vi "Set Active Cursor from Table.vi"(9 "Point":cluster{"horizontal":i32, "vertical":i32}, 10 "Refnums for Resizing and Alignment":T4, 11 "Display State In":T1={"Graph Visible Items"={"Plot Legend"=FALSE, "Scale Legend"=FALSE, "Graph Palette"=FALSE, "Cursor Legend"=FALSE, "X Scrollbar"=FALSE}, "View Table"=FALSE, "Table Visible Items"={"Vertical Scrollbar"=FALSE, "Horizontal Scrollbar"=FALSE, "Row Headers"=FALSE, "Column Headers"=FALSE, "Vertical Lines"=FALSE, "Horizontal Lines"=FALSE}, "Header Font"={"Font Name"="", "Size"=0, "Bold"=FALSE, "Italic"=FALSE, "Underline"=FALSE, "Strikeout"=FALSE, "Color"=0}, "Cell Font"={"Font Name"="", "Size"=0, "Bold"=FALSE, "Italic"=FALSE, "Underline"=FALSE, "Strikeout"=FALSE, "Color"=0}, "Description and Tip..."={"Description"="", "Tip"=""}, "Moveable Splitter Position"=0, "Measurement Cursor Configuration"={"relative to t0"={"enable relative time"=FALSE, "Relative times (DT)"=[], "color"=0}, "range"={"enable range"=FALSE, "T1"=0.0, "T2"=0.0, "Fixed interval (T2-T1)"=0.0, "T1 color"=0, "T2 color"=0, "enable shading"=FALSE}, "periodic"={"enable periodic"=FALSE, "First event (E1)"=0.0, "Number events (Ei)"=0, "Event spacing (s)"=0.0, "First color"=0, "Events color"=0}, "absolute timestamp"={"enable absolute"=FALSE, "Timestamps (TS)"=[], "color"=0}}, "X Increment"=0.0, "X Scale"={"Label Visible"=FALSE, "Label Text"="", "Time Mode"=enum."Relative", "Format String"=""}, "Y Scale"={"Label Visible"=FALSE, "Label Text"="", "Scaling"=enum."Engineering Units", "Format String"=""}, "Colors"={"background"=16777215, "major grid"=8355711, "minor grid"=12632256, "font"=0}, "Cursors"={"List"=[], "Tags"=[]}, "Plots"=[], "Plot Color Wheel"=[3381759, 32768, 982784, 4375295, 13827953, 13457919, 16757522, 4343295, 16728758, 12095254], "registered user events"=variant} caption="State") -> (3 "Display State Out":T1={"Graph Visible Items"={"Plot Legend"=FALSE, "Scale Legend"=FALSE, "Graph Palette"=FALSE, "Cursor Legend"=FALSE, "X Scrollbar"=FALSE}, "View Table"=FALSE, "Table Visible Items"={"Vertical Scrollbar"=FALSE, "Horizontal Scrollbar"=FALSE, "Row Headers"=FALSE, "Column Headers"=FALSE, "Vertical Lines"=FALSE, "Horizontal Lines"=FALSE}, "Header Font"={"Font Name"="", "Size"=0, "Bold"=FALSE, "Italic"=FALSE, "Underline"=FALSE, "Strikeout"=FALSE, "Color"=0}, "Cell Font"={"Font Name"="", "Size"=0, "Bold"=FALSE, "Italic"=FALSE, "Underline"=FALSE, "Strikeout"=FALSE, "Color"=0}, "Description and Tip..."={"Description"="", "Tip"=""}, "Moveable Splitter Position"=0, "Measurement Cursor Configuration"={"relative to t0"={"enable relative time"=FALSE, "Relative times (DT)"=[], "color"=0}, "range"={"enable range"=FALSE, "T1"=0.0, "T2"=0.0, "Fixed interval (T2-T1)"=0.0, "T1 color"=0, "T2 color"=0, "enable shading"=FALSE}, "periodic"={"enable periodic"=FALSE, "First event (E1)"=0.0, "Number events (Ei)"=0, "Event spacing (s)"=0.0, "First color"=0, "Events color"=0}, "absolute timestamp"={"enable absolute"=FALSE, "Timestamps (TS)"=[], "color"=0}}, "X Increment"=0.0, "X Scale"={"Label Visible"=FALSE, "Label Text"="", "Time Mode"=enum."Relative", "Format String"=""}, "Y Scale"={"Label Visible"=FALSE, "Label Text"="", "Scaling"=enum."Engineering Units", "Format String"=""}, "Colors"={"background"=16777215, "major grid"=8355711, "minor grid"=12632256, "font"=0}, "Cursors"={"List"=[], "Tags"=[]}, "Plots"=[], "Plot Color Wheel"=[3381759, 32768, 982784, 4375295, 13827953, 13457919, 16757522, 4343295, 16728758, 12095254], "registered user events"=variant} caption="State")   [LabVIEW 2017, in "Waveforms with Cursors.xctl"]
doc: "Make selected row active cursor and highlight cursor row in table."
uses:
  <vilib>/addons/_XControls/Waveforms with Cursors/Waveforms with Cursors.xctl
  <vilib>/addons/_XControls/Waveforms with Cursors/Controls/State.ctl
  <vilib>/Utility/miscctls.llb/LVFontTypeDef.ctl
  <vilib>/addons/_XControls/Waveforms with Cursors/Controls/Waveform Cursor Configuration.ctl
  <vilib>/addons/_XControls/Waveforms with Cursors/Controls/Refnums Typedef.ctl
  <vilib>/Utility/miscctls.llb/LVPositionTypeDef.ctl
  <vilib>/Utility/miscctls.llb/LVRowAndColumnTypeDef.ctl
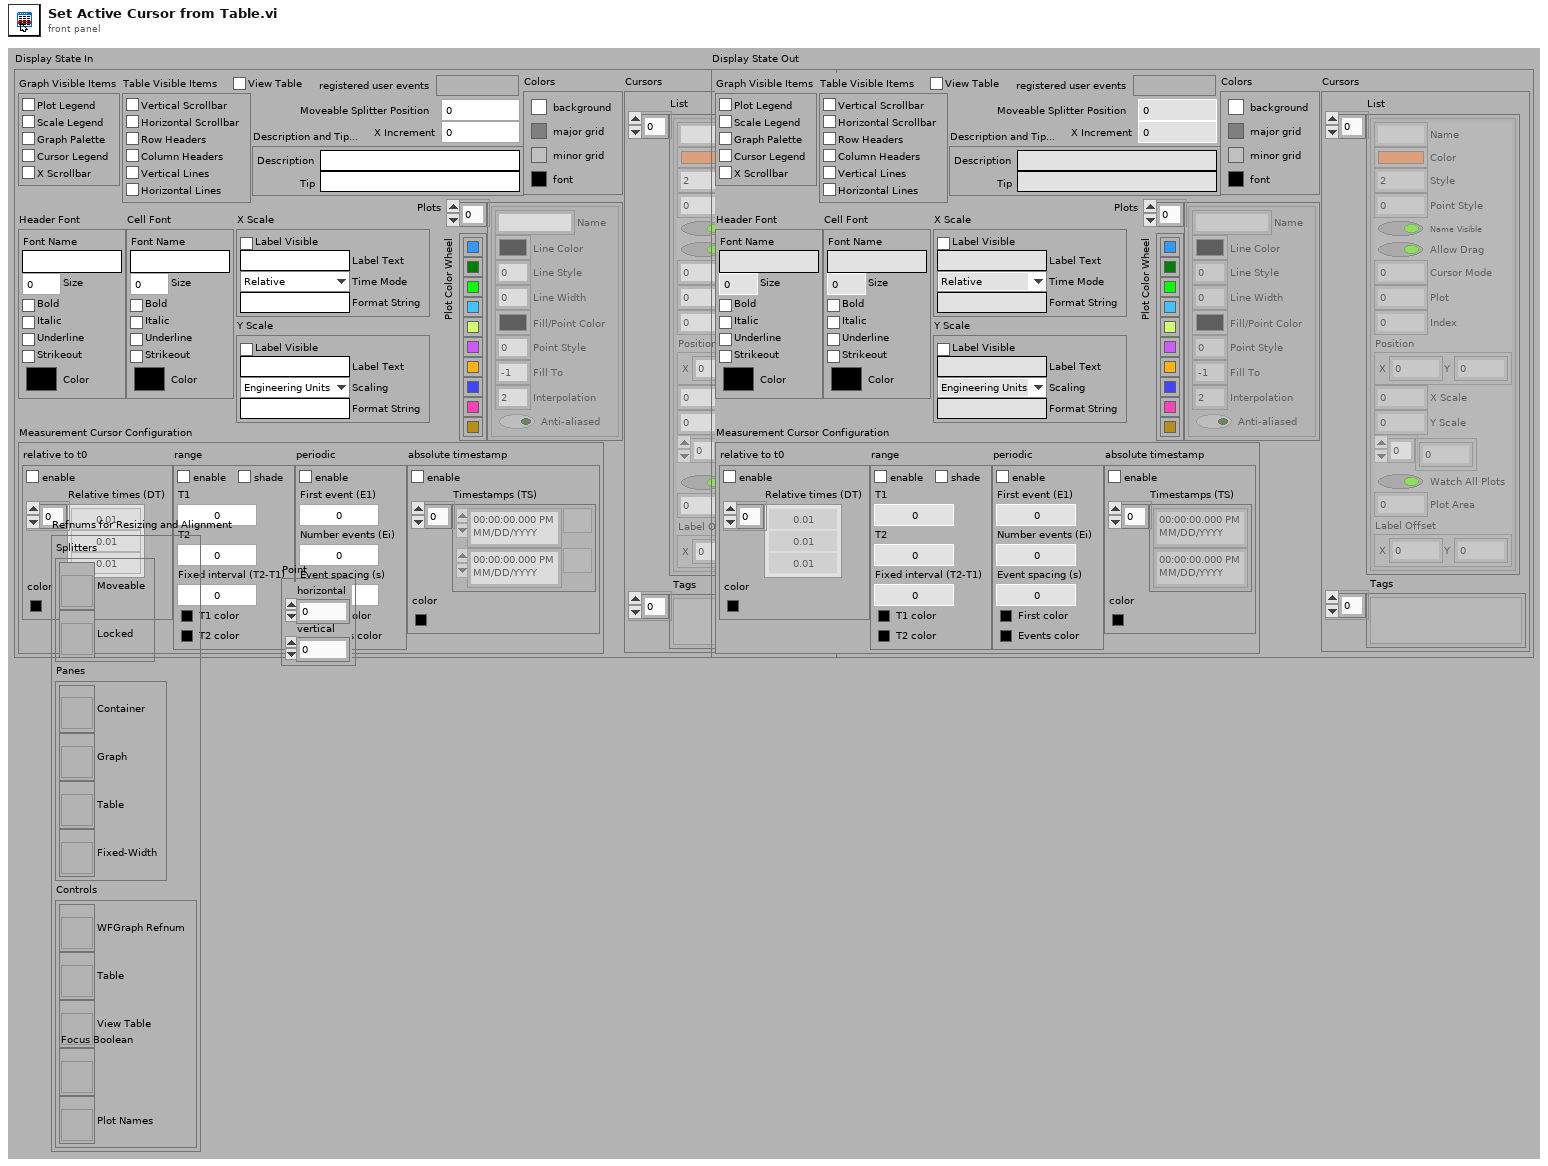
[diagram p1: front panel]
types:
  T1 = typedef "Waveforms with Cursors.xctl/State.ctl" = cluster{"Graph Visible Items":cluster{"Plot Legend":bool, "Scale Legend":bool, "Graph Palette":bool, "Cursor Legend":bool, "X Scrollbar":bool}, "View Table":bool, "Table Visible Items":cluster{"Vertical Scrollbar":bool, "Horizontal Scrollbar":bool, "Row Headers":bool, "Column Headers":bool, "Vertical Lines":bool, "Horizontal Lines":bool}, "Header Font":T2, "Cell Font":T2, "Description and Tip...":cluster{"Description":string, "Tip":string}, "Moveable Splitter Position":i32, "Measurement Cursor Configuration":T3, "X Increment":dbl, "X Scale":cluster{"Label Visible":bool, "Label Text":string, "Time Mode":enum16{"Relative", "Absolute"}, "Format String":string}, "Y Scale":cluster{"Label Visible":bool, "Label Text":string, "Scaling":enum16{"Engineering Units", "Voltage"}, "Format String":string}, "Colors":cluster{"background":u32, "major grid":u32, "minor grid":u32, "font":u32}, "Cursors":cluster{"List":cluster{"Name":string, "Color":u32, "Style":i32, "Point Style":u8, "Name Visible":bool, "Allow Drag":bool, "Cursor Mode":u32, "Plot":i32, "Index":i32, "Position":cluster{"X":dbl, "Y":dbl}, "X Scale":u32, "Y Scale":u32, "Watch Plots":i32[], "Watch All Plots":bool, "Plot Area":i32, "Label Offset":cluster{"X":dbl, "Y":dbl}}[], "Tags":variant[]}, "Plots":cluster{"Name":string, "Line Color":u32, "Line Style":u8, "Line Width":u8, "Fill/Point Color":u32, "Point Style":u8, "Fill To":i16, "Interpolation":u8, "Anti-aliased":bool}[], "Plot Color Wheel":u32[], "registered user events":variant}
  T2 = typedef "LVFontTypeDef.ctl" = cluster{"Font Name":string, "Size":u16, "Bold":bool, "Italic":bool, "Underline":bool, "Strikeout":bool, "Color":u32}
  T3 = typedef "Waveforms with Cursors.xctl/Waveform Cursor Configuration.ctl" = cluster{"relative to t0":cluster{"enable relative time":bool, "Relative times (DT)":dbl[], "color":u32}, "range":cluster{"enable range":bool, "T1":dbl, "T2":dbl, "Fixed interval (T2-T1)":dbl, "T1 color":u32, "T2 color":u32, "enable shading":bool}, "periodic":cluster{"enable periodic":bool, "First event (E1)":dbl, "Number events (Ei)":i32, "Event spacing (s)":dbl, "First color":u32, "Events color":u32}, "absolute timestamp":cluster{"enable absolute":bool, "Timestamps (TS)":timestamp[], "color":u32}}
  T4 = typedef "Waveforms with Cursors.xctl/Refnums Typedef.ctl" = cluster{"Splitters":cluster{"Moveable":refnum<vi>, "Locked":refnum<vi>}, "Panes":cluster{"Container":refnum<vi>, "Graph":refnum<vi>, "Table":refnum<vi>, "Fixed-Width":refnum<vi>}, "Controls":cluster{"WFGraph Refnum":refnum<vi>, "Table":refnum<vi>, "View Table":refnum<vi>, "Focus Boolean":refnum<vi>, "Plot Names":refnum<vi>}}
  T5 = typedef "LVPositionTypeDef.ctl" = cluster{"Left":i32, "Top":i32}
  T6 = typedef "LVRowAndColumnTypeDef.ctl" = cluster{"Row":i32, "Column":i32}
  T7 = cluster{"Name":string, "Color":u32, "Style":i32, "Point Style":u8, "Name Visible":bool, "Allow Drag":bool, "Cursor Mode":u32, "Plot":i32, "Index":i32, "Position":cluster{"X":dbl, "Y":dbl}, "X Scale":u32, "Y Scale":u32, "Watch Plots":i32[], "Watch All Plots":bool, "Plot Area":i32, "Label Offset":cluster{"X":dbl, "Y":dbl}}[]
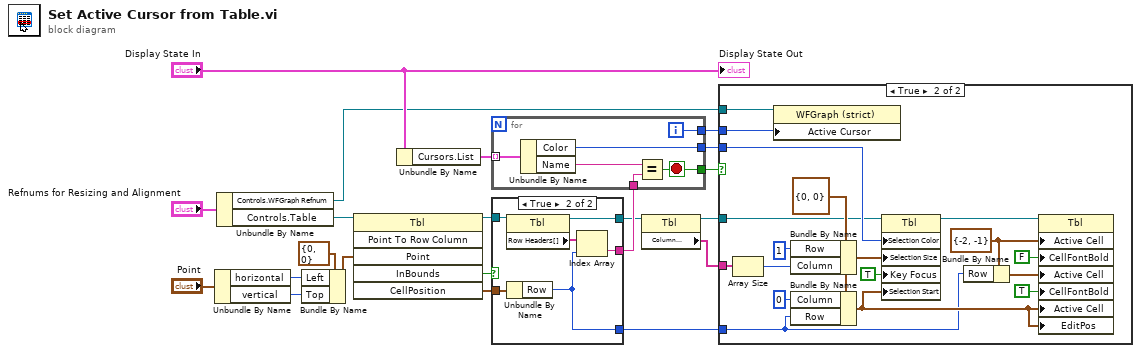
[diagram p0: block diagram]
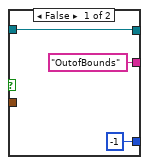
[diagram p3: hidden frame]
diagram:
  n1 = Unbundle By Name("Point") -> ("horizontal"=w9:i32, "vertical"=w8:i32)
  n2 = Unbundle By Name("Refnums for Resizing and Alignment") -> ("Controls.WFGraph Refnum"=w7:refnum<vi>, "Controls.Table"=w16:refnum<vi>)
  n3 = Bundle By Name(cluster=T5 {"Left"=0, "Top"=0} ("Point"), "Left"=w9, "Top"=w8) -> (w10:T5)
  n4 = invoke class="Tbl" method="Point To Row Column"(reference=w16, "Point"=w10) -> (reference out=w17:refnum<vi>, "InBounds"=w15:bool, "CellPosition"=w1:T6)  [unwired: 4 in, 3 out]
  n5 = Unbundle By Name("Display State In") -> ("Cursors.List"=w18:T7)
  n6 = case shown="True" w15 {
    tunnel: w1 -> [_ w30]
    tunnel: w17 -> [w23 w29]
    tunnel: ["OutofBounds" w27] -> w19
    tunnel: [w23 w26] -> w4
    tunnel: [-1 ("Row") w25] -> w6
    frame False {
    }
    frame True {
      n7 = property class="Tbl"(reference=w29) -> (reference out=w26:refnum<vi>, "Row Headers[]"=w28:string[])  [unwired: 1 in, 1 out]
      n8 = Unbundle By Name(w30) -> ("Row"=w25:i32)
      n9 = Index Array(array=w28, index=w25) -> (element=w27:string)
    }
  }
  n10 = for {
    tunnel: w18 -> [w33] mode=indexing
    tunnel: w19 -> [w36]
    tunnel: [w35] -> w20
    tunnel: [w34] -> w21
    tunnel: [w32] -> w5
    i -> [w34]
    stop <- w35 stop-if-true
    n11 = Unbundle By Name(w33) -> ("Color"=w32:u32, "Name"=w31:string)
    n12 = Equal?(x=w31, y=w36) -> (x = y?=w35:bool)
  }
  n13 = property class="Tbl"(reference=w4) -> (reference out=w3:refnum<vi>, "Column Headers[]"=w2:string[])  [unwired: 1 in, 1 out]
  n14 = case shown="True" w20 {
    tunnel: w7 -> [_ w54]
    tunnel: w21 -> [_ w53]
    tunnel: w6 -> [_ w37]
    tunnel: w5 -> [_ w48]
    tunnel: w3 -> [_ w47]
    tunnel: w2 -> [_ w46]
    frame False {
    }
    frame True {
      w42 = T6 {"Row"=-2, "Column"=-1} ("Active Cell:Active Cell")
      w49 = T6 {"Row"=0, "Column"=0} ("Selection Size")
      n15 = Array Size(array=w46) -> (size(s)=w44:i32)
      n16 = property class="WFGraph (strict)"(reference=w54, "Active Cursor"=w53) -> ()  [unwired: 1 in, 2 out]
      n17 = Bundle By Name(cluster=w49, "Row"=1, "Column"=w44) -> (w51:T6)
      n18 = Bundle By Name(cluster=w49, "Column"=0, "Row"=w37) -> (w38:T6)
      n19 = property class="Tbl"(reference=w47, "Selection Color"=w48, "Selection Size"=w51, "Key Focus"=TRUE, "Selection Start"=w38) -> (reference out=w39:refnum<vi>)  [unwired: 1 in, 1 out]
      n20 = Bundle By Name(cluster=w42, "Row"=w37) -> (w43:T6)
      n21 = property class="Tbl"(reference=w39, "Active Cell"=w42, "CellFontBold"=FALSE ("Active Cell:Cell Font:Bold"), "Active Cell"=w43, "CellFontBold"=TRUE ("Active Cell:Cell Font:Bold"), "Active Cell"=w38, "EditPos"=w38) -> ()  [unwired: 1 in, 2 out]
    }
  }
  "Display State Out" <- "Display State In"
